vi "Update Status Log.vi"(8 "error in (no error)":errorcluster, 9 "Status List":string[](array[string]), 10 "Names":string[](array[string]), 11 "Chat Window Model in":refnum<class "Chat Window Model.lvclass">) -> (0 "error out":errorcluster, 3 "Chat Window Model out":refnum<class "Chat Window Model.lvclass">)   [LabVIEW 2015, in "Chat Window Model.lvlib" / "Chat Window Model.lvclass"]
uses:
  Chat Window Model.lvclass
  Chat Window UI Controller/Chat Window UI Controller Messages/Update Status List Msg/Update Status List Msg.lvclass
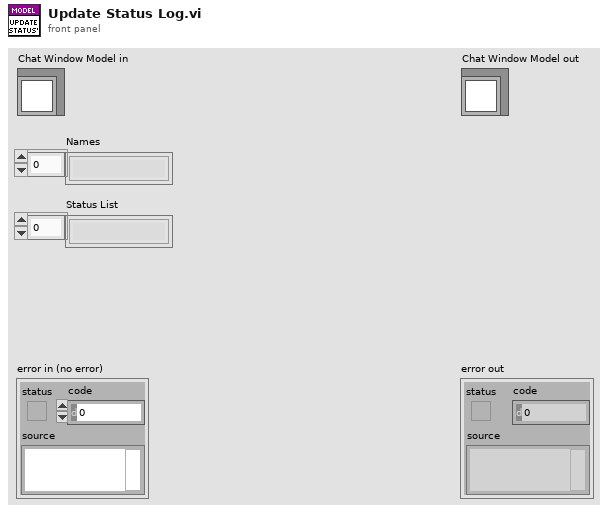
[diagram p1: front panel]
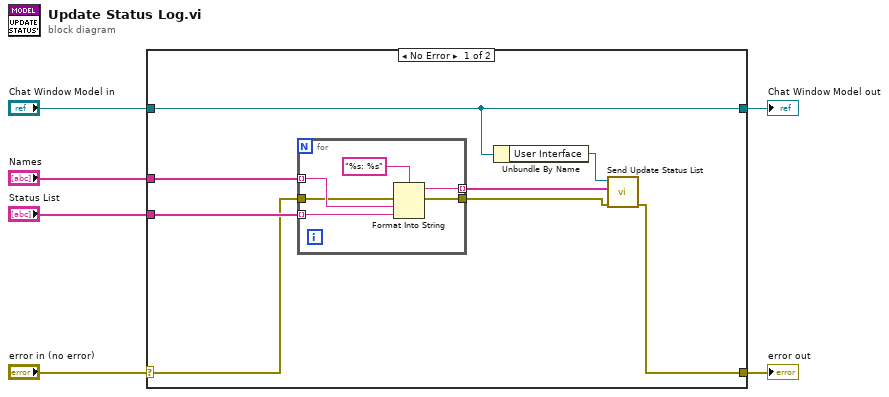
[diagram p0: block diagram]
diagram:
  n1 = case shown="No Error" "error in (no error)" {
    selector: "error in (no error)" -> [w7 w22]
    tunnel: [w9 w22] -> w5
    tunnel: [w11 w21] -> w3
    tunnel: "Chat Window Model in" -> [w11 w21]
    tunnel: "Names" -> [w14 _]
    tunnel: "Status List" -> [w13 _]
    frame No Error {
      n2 = for {
        tunnel: w14 -> [w19] mode=indexing
        tunnel: w13 -> [w18] mode=indexing
        tunnel: [w17] -> w12 mode=indexing
        tunnel: [w16] -> w8
        tunnel: w7 -> [w15]
        n3 = Format Into String(format string="%s: %s", error in=w15, w19, w18) -> (resulting string=w17:string, error out=w16:errorcluster)  [unwired: 1 in]
      }
      n4 = Unbundle By Name(w11) -> ("User Interface"=w10:refnum<class "Message Enqueuer.lvclass">)
      n5 = call "Send Update Status List.vi"("error in (no error)"=w8, "Status List"=w12, "Message Enqueuer"=w10) -> ("error out"=w9:errorcluster)  [unwired: 7 in, 1 out]
    }
    frame Error {
    }
  }
  "error out" <- w5
  "Chat Window Model out" <- w3
